vi "Boiler Running.vi"(6 "Boiler Simulation Controls":T1 {"Flame Sensor Value (%)" min=0.0 max=100.0 scale=0.0..100.0}, 8 "error in (no error)":errorcluster, 9 "Boiler Controls":T2 {"Fuel Valve Position" min=0.0 max=100.0 scale=0.0..100.0 scale format="%.2f"}, 10 "Indicator states in":T4 {"Time Count" format="%.2g"}, 11 "Runtime statuses in":T3) -> (0 "error out":errorcluster, 2 "Indicator states out":T4 {"Time Count" format="%.2g"}, 3 "Runtime statuses out":T3)   [LabVIEW 2014]
doc: "Boiler running state. Checks if conditions are valid for boiler to run, othervise starts shutdown sequence"
uses:
  Controls/Boiler Status Indicators.ctl
  Controls/Boiler runtime status indicators.ctl
  Controls/Boiler Controls.ctl
  Controls/Boiler Simulation Controls.ctl
  Controls/Log file FGV action enum.ctl
  Controls/Log event enum.ctl
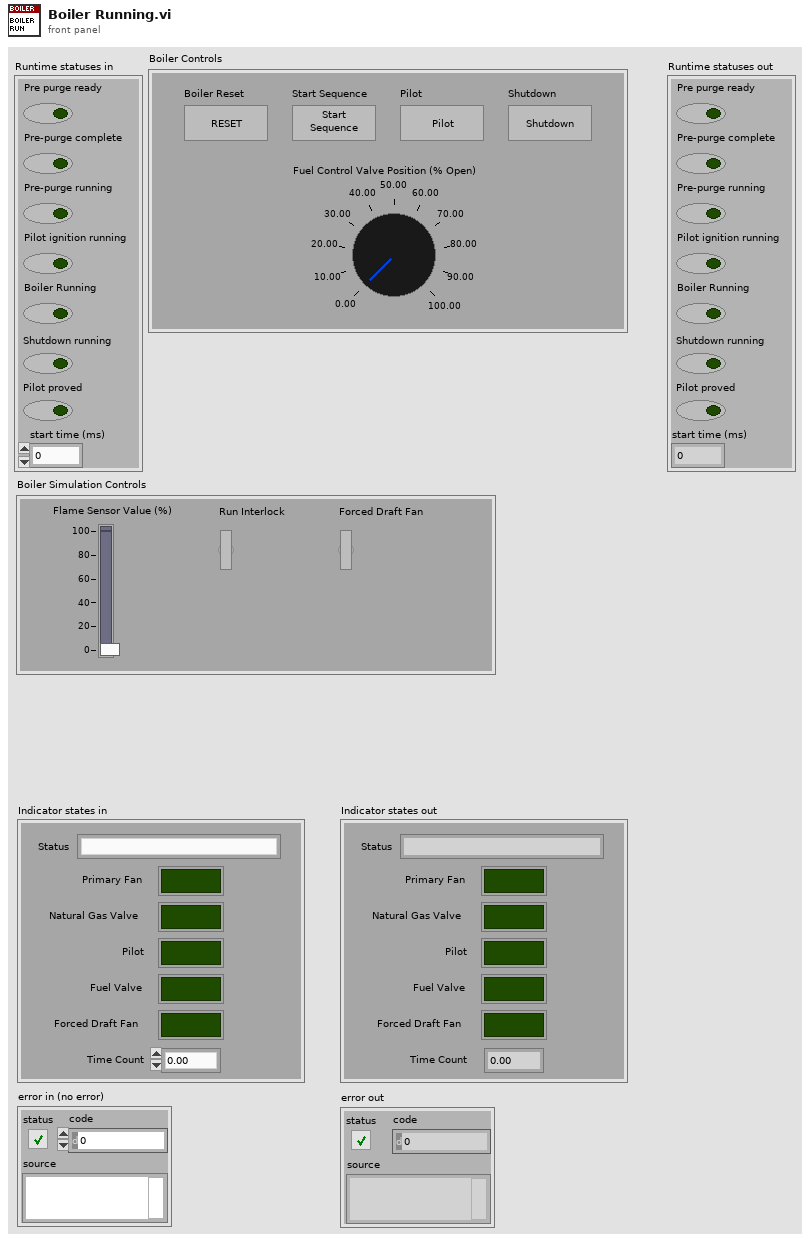
[diagram p1: front panel]
types:
  T1 = typedef "Boiler Simulation Controls.ctl" = cluster{"Flame Sensor Value (%)":dbl, "Run Interlock":bool, "Forced Draft Fan":bool}
  T2 = typedef "Boiler Controls.ctl" = cluster{"Boiler Reset":bool, "Start Sequence":bool, "Pilot":bool, "Shutdown":bool, "Fuel Valve Position":dbl}
  T3 = typedef "Boiler runtime status indicators.ctl" = cluster{"Pre purge ready":bool, "Pre-purge complete":bool, "Pre-purge running":bool, "Pilot ignition running":bool, "Boiler Running":bool, "Shutdown running":bool, "Pilot proved":bool, "start time (ms)":u32}
  T4 = typedef "Boiler Status Indicators.ctl" = cluster{"Status":string, "Primary Fan":bool, "Natural Gas Valve":bool, "Pilot":bool, "Fuel Valve":bool, "Forced Draft Fan":bool, "Time Count":dbl}
  T5 = typedef "Log event enum.ctl" = enum16{"Boiler Initialized", "Boiler Ready", "Start Pre-Purge", "Pre-Purge Complete", "Pilot ON", "Pilot proved", "Forced Draft Fan ON", "Boiler Running", "Start Shutdown Purge", "Shutdown Purge Complete"}
  T6 = typedef "Log file FGV action enum.ctl" = enum16{"open log file", "log event", "close log file"}
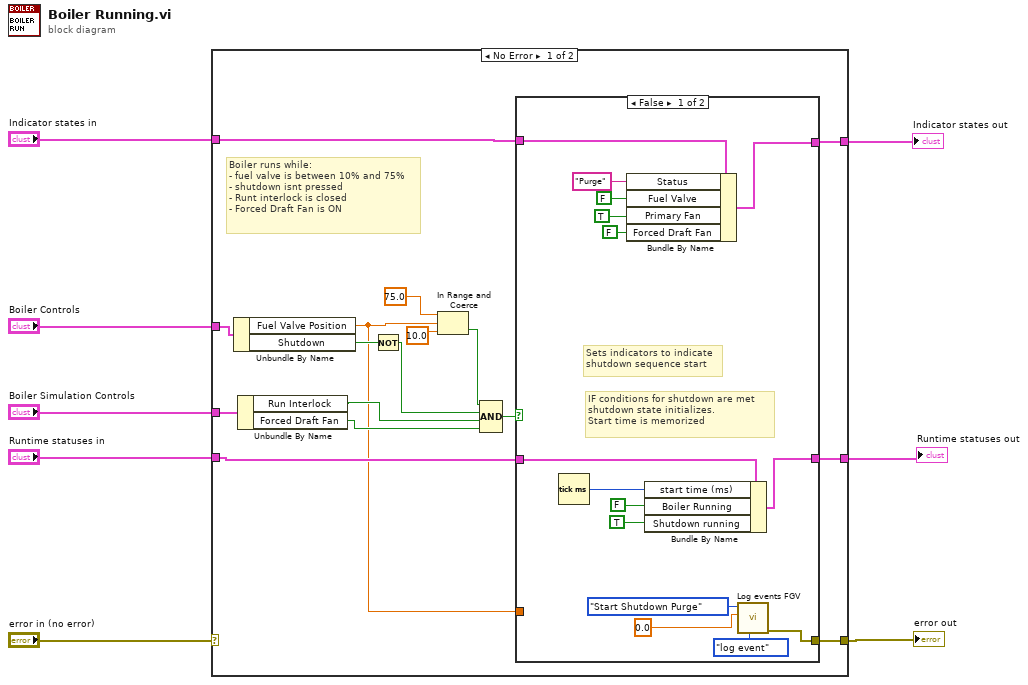
[diagram p0: block diagram]
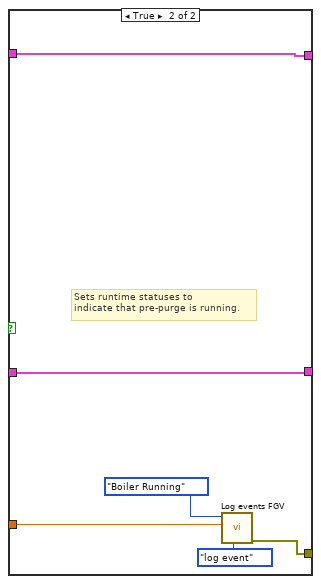
[diagram p2: hidden frame]
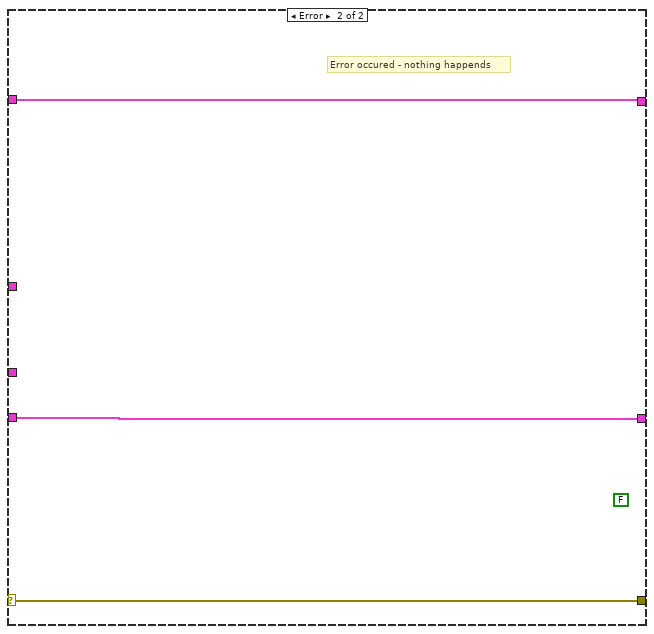
[diagram p3: hidden frame]
diagram:
  n1 = case shown="No Error" "error in (no error)" {
    selector: "error in (no error)" -> [_ w48]
    tunnel: [w10 w48] -> w7
    tunnel: "Runtime statuses in" -> [w21 w46]
    tunnel: "Indicator states in" -> [w23 w47]
    tunnel: [w22 w47] -> w4
    tunnel: [w20 w46] -> w3
    tunnel: "Boiler Controls" -> [w19 _]
    tunnel: "Boiler Simulation Controls" -> [w14 _]
    frame No Error {
      # "Boiler runs while:\n- fuel valve is between 10% and 75%\n- shutdown isnt pressed\n- Runt interlock is closed\n- Forced Draft Fan is ON"
      n2 = Unbundle By Name(w19) -> ("Fuel Valve Position"=w9:dbl, "Shutdown"=w15:bool)
      n3 = Unbundle By Name(w14) -> ("Run Interlock"=w13:bool, "Forced Draft Fan"=w12:bool)
      n4 = Not(x=w15) -> (.not. x?=w11:bool)
      n5 = In Range and Coerce(upper limit=75.0 ("lower limit"), x=w9, lower limit=10.0) -> (In Range?=w18:bool)  [unwired: 1 out]
      n6 = Compound Arithmetic op=AND(w18, w11, w13, w12) -> (w24:bool)
      n7 = case shown="False" w24 {
        tunnel: w23 -> [w35 w44]
        tunnel: [w32 w44] -> w22
        tunnel: w21 -> [w39 w45]
        tunnel: [w38 w45] -> w20
        tunnel: [w26 w41] -> w10
        tunnel: w9 -> [_ w40]
        frame False {
          # "Sets indicators to indicate\nshutdown sequence start"
          # "IF conditions for shutdown are met\nshutdown state initializes.\nStart time is memorized"
          n8 = Tick Count (ms)() -> (millisecond timer value=w30:u32)
          n9 = Bundle By Name(cluster=w35, "Status"="Purge", "Fuel Valve"=FALSE, "Primary Fan"=TRUE, "Forced Draft Fan"=FALSE) -> (w32:T4)
          n10 = Bundle By Name(cluster=w39, "start time (ms)"=w30, "Boiler Running"=FALSE, "Shutdown running"=TRUE) -> (w38:T3)
          n11 = call "Log events FGV.vi"("action"=Log_file_FGV_action_enum."log event", "Event data"=0.0 ("lower limit"), "Log event"=Log_event_enum."Start Shutdown Purge") -> ("error out"=w26:errorcluster)  [unwired: 8 in]
        }
        frame True {
          # "Sets runtime statuses to\nindicate that pre-purge is running."
          n12 = call "Log events FGV.vi"("action"=Log_file_FGV_action_enum."log event", "Event data"=w40, "Log event"=Log_event_enum."Boiler Running") -> ("error out"=w41:errorcluster)  [unwired: 8 in]
        }
      }
    }
    frame Error {
      (unwired) FALSE
      # "Error occured - nothing happends"
    }
  }
  "Indicator states out" <- w4
  "error out" <- w7
  "Runtime statuses out" <- w3
